vi "Base64_EncodeAnything.vi"(8 "error in (no error)":errorcluster, 11 "Variant":variant) -> (0 "error out":errorcluster, 2 "Encoded Payload":string, 3 "Variant dup":variant)   [LabVIEW 2013, in "Serializer.Base64.lvclass"]
uses:
  Serializer.Base64.lvclass
  <vilib>/LabVIEW Open Source Project/OpenSerializer/Serializer/Serializer.lvclass
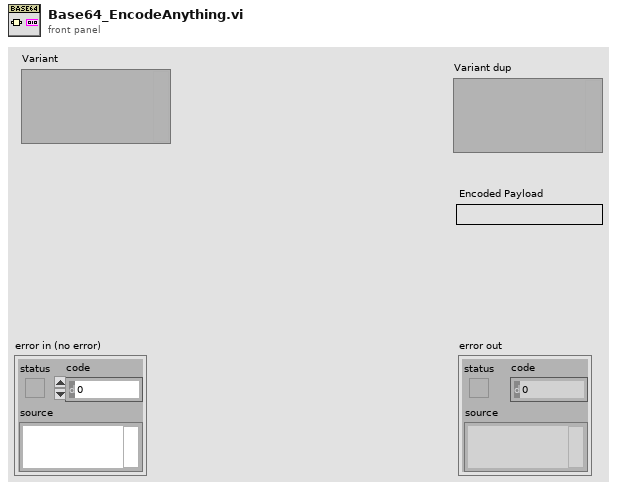
[diagram p1: front panel]
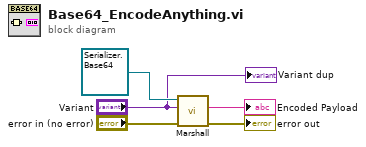
[diagram p0: block diagram]
diagram:
  n1 = call <vilib>:"Marshall.vi"("error in (no error)"="error in (no error)", "Variant"="Variant", "Serializer in"=refnum<class "Serializer.Base64.lvclass"> refnum ("Serializer.Base64 in")) -> ("error out"=→"error out":errorcluster, "String"=→"Encoded Payload":string)  [unwired: 6 in, 1 out]
  "Variant dup" <- "Variant"
